vi "Configure Tester Dialog.vi"(8 "error in":errorcluster, 11 "Potting Procedure In":refnum<class "Potting Procedure.lvclass">) -> (0 "error out":errorcluster, 2 "Canceled":bool, 3 "Potting Procedure Out":refnum<class "Potting Procedure.lvclass">)   [LabVIEW 2011]
uses:
  UI typedefs/Chuck Control.ctl
  UI typedefs/Chuck Slot Control.ctl
  Procedure Classes/Potting Procedure/Potting Procedure.lvclass
  Shared Components/WorkTable Class/WorkTable Class.lvclass
  Procedure Classes/Potting Procedure/Type Definitions/Configure Tester.ctl
panel:
  in  "Module Chuck 5":T1
  in  "Module Chuck 4":T1
  in  "Module Chuck 3":T1
  in  "Module Chuck 2":T1
  in  "Module Chuck 1":T1
  in  "OK Button":bool
  in  "Cancel Button":bool
  # "Click inside the boxes to indicate whether\na slot is populated.\n\nFor each populated chuck enter the serial\nnumber in the provided text field."
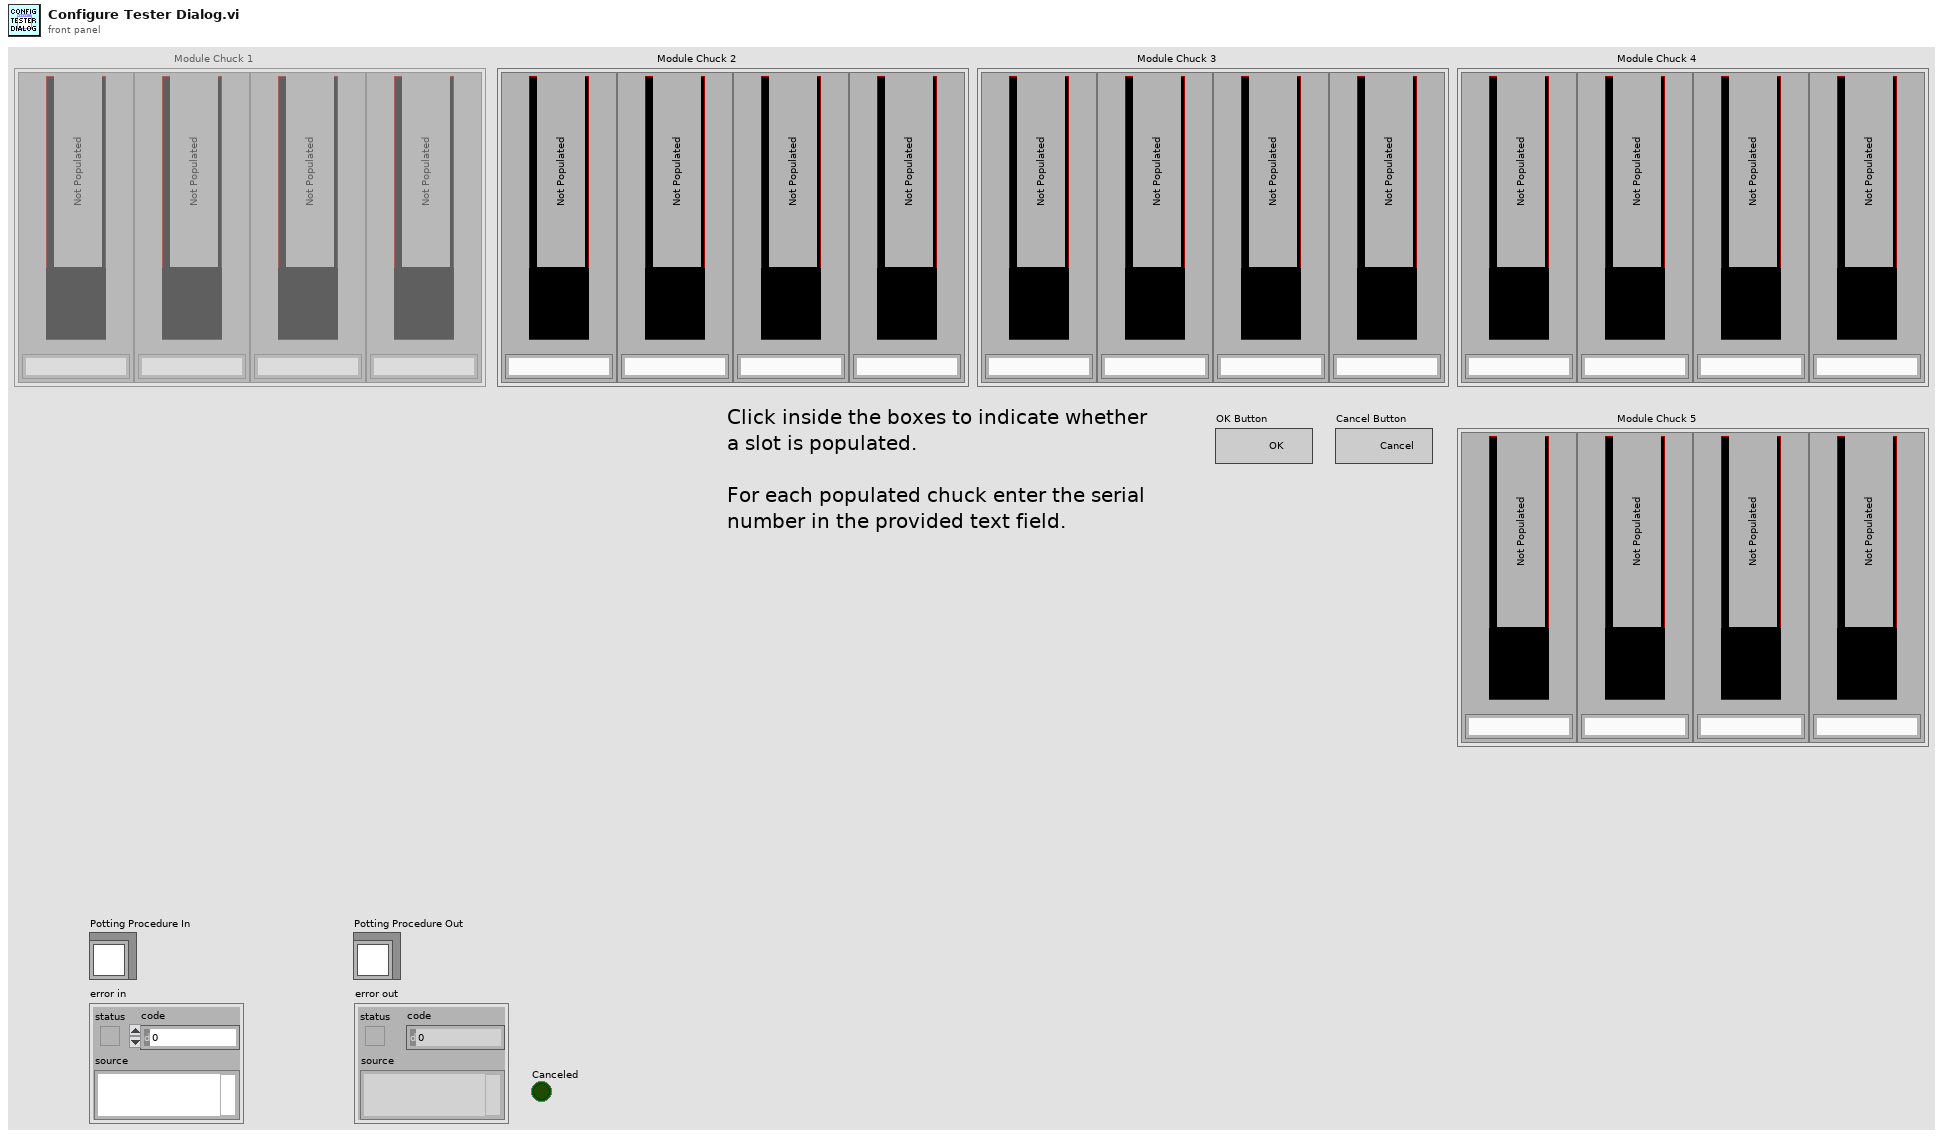
[diagram p1: front panel]
types:
  T1 = typedef "Chuck Control.ctl" = cluster{"Slot 1":T2, "Slot 2":T2, "Slot 3":T2, "Slot 4":T2}
  T2 = typedef "Chuck Slot Control.ctl" = cluster{"Slot Populated":bool, "S/N":string}
  T3 = enum8{"Enabled", "Disabled", "Disabled and Grayed Out"}
  T4 = enum16{"Empty", "Unglued", "Stamped", "PartOnTop", "Weighted", "Unpotted", "Potted"}
  T5 = typedef "Worktable_Module Slot.ctl" = cluster{"Slot State":enum16{"Empty", "Unglued", "Stamped", "PartOnTop", "Weighted", "Unpotted", "Potted"}, "BBM Type":enum16{"None", "BBM", "GlassSlide"}, "HDI Type":enum16{"None", "HDI", "Polyimide"}, "Vacuum Channel":u8, "Location/Orientation BBM":T6, "Location/Orientation HDI":T6, "S/N":string}
  T6 = typedef "Position_Orientation.ctl" = cluster{"Center":refnum<class "Vec3d Class.lvclass">, "Orientation":refnum<class "Orient3d Class.lvclass">}
  T7 = typedef "Configure Tester.ctl" = cluster{"Has Been Run?":bool}
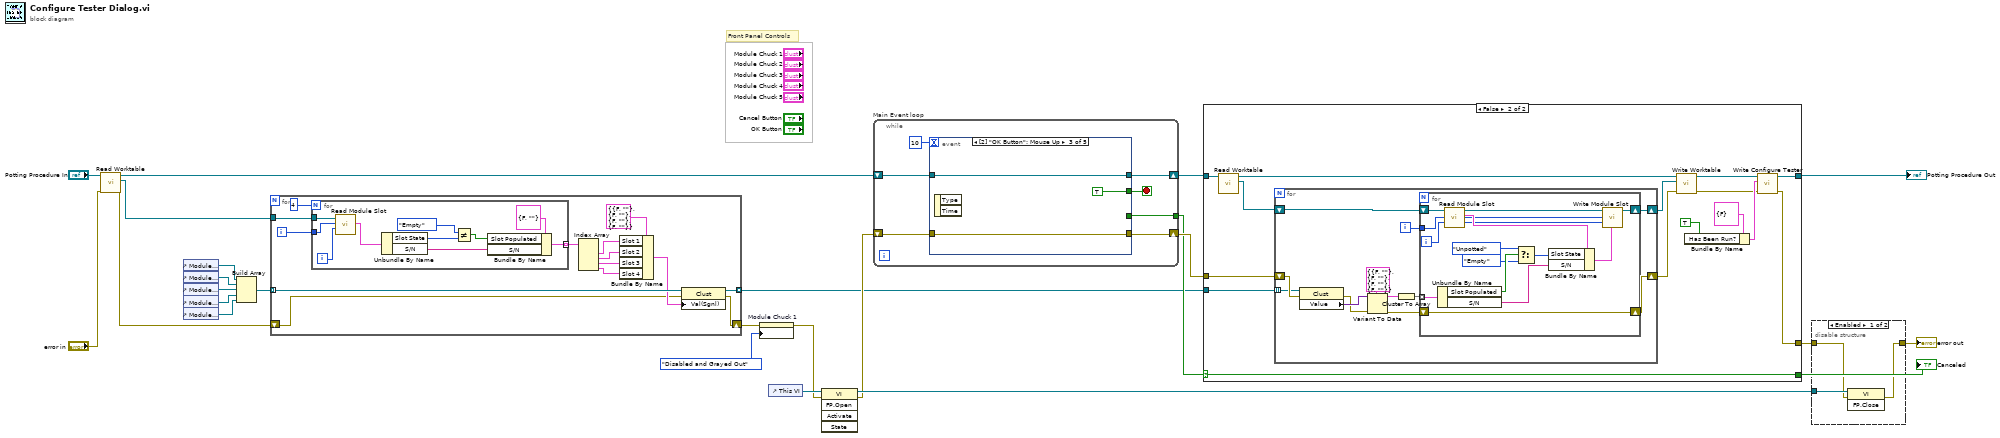
[diagram p0: block diagram]
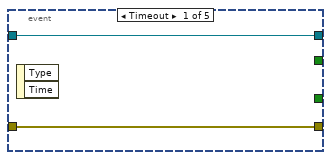
[diagram p4: hidden frame]
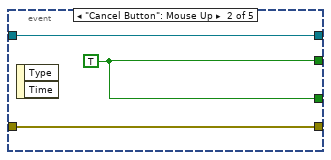
[diagram p5: hidden frame]
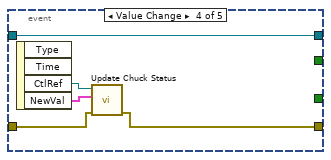
[diagram p6: hidden frame]
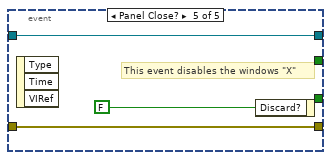
[diagram p7: hidden frame]
diagram:
  # "Front Panel Controls"
  n1 = call-dynamic "Read Worktable.vi"("error in"="error in", "Potting Procedure in"="Potting Procedure In") -> ("error out"=w4:errorcluster, "WorkTable out"=w5:refnum<class "WorkTable Class.lvclass">, "Potting Procedure out"=w17:refnum<class "Potting Procedure.lvclass">)  [unwired: 7 in]
  n2 = control-ref of="Module Chuck 1"() -> (w10:refnum<vi>)
  n3 = control-ref of="Module Chuck 2"() -> (w9:refnum<vi>)
  n4 = control-ref of="Module Chuck 3"() -> (w8:refnum<vi>)
  n5 = control-ref of="Module Chuck 4"() -> (w7:refnum<vi>)
  n6 = control-ref of="Module Chuck 5"() -> (w6:refnum<vi>)
  n7 = Build Array(w10, w9, w8, w7, w6) -> (w2:refnum<vi>[])
  n8 = for {
    tunnel: w2 -> [w32] mode=indexing
    shift-right: [w30] -> w3
    shift-left: w4 -> [w29]
    tunnel: w5 -> [w27]
    tunnel: [w28] -> w1 mode=indexing
    i -> [w26]
    n9 = for {
      N: 4 -> [_]
      tunnel: [w46] -> w37 mode=indexing
      tunnel: w27 -> [w43]
      tunnel: w26 -> [w41]
      i -> [w42]
      n10 = call-dynamic "Read Module Slot.vi"("slot"=w42, "chuck"=w41, "WorkTable in"=w43) -> ("Module Slot"=w40:T5)  [unwired: 6 in, 2 out]
      n11 = Unbundle By Name(w40) -> ("Slot State"=w45:T4, "S/N"=w44:string)
      n12 = Not Equal?(x=T4."Empty" ("BBM Slot State"), y=w45) -> (x != y?=w47:bool)
      n13 = Bundle By Name(cluster=T2 {"Slot Populated"=FALSE, "S/N"=""} ("Slot 1"), "Slot Populated"=w47, "S/N"=w44) -> (w46:T2)
    }
    n14 = Index Array(array=w37) -> (element #1=w36:T2, element #2=w35:T2, element #3=w34:T2, element #4=w33:T2)  [unwired: 4 in]
    n15 = Bundle By Name(cluster=T1 {"Slot 1"={"Slot Populated"=FALSE, "S/N"=""}, "Slot 2"={"Slot Populated"=FALSE, "S/N"=""}, "Slot 3"={"Slot Populated"=FALSE, "S/N"=""}, "Slot 4"={"Slot Populated"=FALSE, "S/N"=""}} ("BBM Chuck 1"), "Slot 1"=w36, "Slot 2"=w35, "Slot 3"=w34, "Slot 4"=w33) -> (w31:T1)
    n16 = property class="Clust"(reference=w32, error in=w29, "Val(Sgnl)"=w31) -> (reference out=w28:refnum<vi>, error out=w30:errorcluster)
  }
  n17 = property on="Module Chuck 1" class="Clust"(error in=w3, "DisabledEnum"=T3."Disabled and Grayed Out" ("Disabled")) -> (error out=w12:errorcluster)  [unwired: 1 in, 1 out]
  n18 = control-ref of="This VI"() -> (w25:refnum<vi>)
  n19 = invoke class="VI" method="FP.Open"(reference=w25, error in=w12) -> (reference out=w24:refnum<vi>, error out=w22:errorcluster)  [unwired: 3 in, 3 out]
  n20 = while "Main Event loop" {
    tunnel: [w52] -> w14
    shift-right: [w50] -> w20
    shift-left: w17 -> [w51]
    shift-right: [w54] -> w16
    shift-left: w22 -> [w53]
    stop <- w55 stop-if-true
    n21 = event shown="[2] \"OK Button\": Mouse Up" {
      selector: _ -> [_ _ _ _ _]
      dyn-events: _ -> [_ _ _ _ _]
      timeout: 10 -> [_ _ _ _ _]
      tunnel: [_ w60 TRUE _ _] -> w55
      tunnel: [w58 w61 w64 w65 w71] -> w54
      tunnel: w53 -> [w58 w61 w64 w68 w71]
      tunnel: [_ w60 _ _ _] -> w52
      tunnel: w51 -> [w57 w59 w62 w66 w70]
      tunnel: [w57 w59 w62 w66 w70] -> w50
      event Timeout {
        n22 = event-data() -> ()  [unwired: 1 in, 2 out]
      }
      event "Cancel Button": Mouse Up {
        w60 = TRUE
        n23 = event-data() -> ()  [unwired: 1 in, 2 out]
      }
      event "OK Button": Mouse Up {
        n24 = event-data() -> ()  [unwired: 1 in, 2 out]
      }
      event Value Change {
        n25 = event-data() -> ("CtlRef"=w69:refnum<vi>, "NewVal"=w67:T1)  [unwired: 1 in, 2 out]
        n26 = call "Update Chuck Status.vi"("error in"=w68, "Chuck Value"=w67, "Chuck Reference In"=w69) -> ("error out"=w65:errorcluster)  [unwired: 8 in]
      }
      event Panel Close? {
        # "This event disables the windows \"X\""
        n27 = event-data() -> ()  [unwired: 1 in, 3 out]
        n28 = event-data("Discard?"=FALSE) -> ()  [unwired: 1 in, 1 out]
      }
    }
  }
  n29 = case shown="False" w14 {
    selector: w14 -> [w73 w85]
    tunnel: w20 -> [w75 w84]
    tunnel: [w75 w90] -> w19
    tunnel: w16 -> [w74 w77]
    tunnel: [w74 w87] -> w15
    tunnel: [w73 w85] -> w11
    tunnel: w1 -> [_ w76]
    frame True {
    }
    frame False {
      n30 = call-dynamic "Read Worktable.vi"("Potting Procedure in"=w84) -> ("WorkTable out"=w83:refnum<class "WorkTable Class.lvclass">, "Potting Procedure out"=w82:refnum<class "Potting Procedure.lvclass">)  [unwired: 8 in, 1 out]
      n31 = for {
        shift-right: [w97] -> w78
        shift-left: w83 -> [w99]
        shift-right: [w95] -> w79
        shift-left: w77 -> [w94]
        tunnel: w76 -> [w91] mode=indexing
        i -> [w98]
        n32 = property class="Clust"(reference=w91, error in=w94) -> (error out=w92:errorcluster, "Value"=w93:variant)  [unwired: 1 out]
        n33 = Variant To Data(error in=w92, type=T1 {"Slot 1"={"Slot Populated"=FALSE, "S/N"=""}, "Slot 2"={"Slot Populated"=FALSE, "S/N"=""}, "Slot 3"={"Slot Populated"=FALSE, "S/N"=""}, "Slot 4"={"Slot Populated"=FALSE, "S/N"=""}} ("BBM Chuck 1"), Variant=w93) -> (data=w101:T1, error out=w96:errorcluster)
        n34 = Cluster To Array(cluster=w101) -> (array=w100:T2[])
        n35 = for {
          tunnel: w100 -> [w116] mode=indexing
          tunnel: w98 -> [w108]
          shift-right: [w106] -> w97
          shift-left: w99 -> [w104]
          shift-right: [w105] -> w95
          shift-left: w96 -> [w105]
          i -> [w109]
          n36 = Unbundle By Name(w116) -> ("Slot Populated"=w114:bool, "S/N"=w115:string)
          n37 = call-dynamic "Read Module Slot.vi"("slot"=w109, "chuck"=w108, "WorkTable in"=w104) -> ("Module Slot"=w110:T5, "WorkTable out"=w103:refnum<class "WorkTable Class.lvclass">)  [unwired: 6 in, 1 out]
          n38 = Select(t=T4."Unpotted" ("BBM Slot State"), s=w114, f=T4."Empty" ("BBM Slot State")) -> (s? t:f=w111:T4)
          n39 = Bundle By Name(cluster=w110, "Slot State"=w111, "S/N"=w115) -> (w107:T5)
          n40 = call-dynamic "Write Module Slot.vi"("Module Slot"=w107, "slot"=w109, "chuck"=w108, "WorkTable in"=w103) -> ("WorkTable out"=w106:refnum<class "WorkTable Class.lvclass">)  [unwired: 6 in, 1 out]
        }
      }
      n41 = call-dynamic "Write Worktable.vi"("error in"=w79, "WorkTable in"=w78, "Potting Procedure in"=w82) -> ("error out"=w80:errorcluster, "Potting Procedure out"=w81:refnum<class "Potting Procedure.lvclass">)  [unwired: 7 in]
      n42 = Bundle By Name(cluster=T7 {"Has Been Run?"=FALSE} ("Configure Tester"), "Has Been Run?"=TRUE) -> (w88:T7)
      n43 = call-dynamic "Write Configure Tester.vi"("error in (no error)"=w80, "Configure Tester"=w88, "Potting Procedure in"=w81) -> ("error out"=w87:errorcluster, "Potting Procedure out"=w90:refnum<class "Potting Procedure.lvclass">)  [unwired: 7 in]
    }
  }
  "Canceled" <- w11
  "Potting Procedure Out" <- w19
  n44 = disable-structure shown="Enabled" {
    disable-tunnel: w24 -> [w119 _]
    disable-tunnel: [w118 w120] -> w23
    disable-tunnel: w15 -> [w117 w120]
    frame Enabled {
      n45 = invoke class="VI" method="FP.Close"(reference=w119, error in=w117) -> (error out=w118:errorcluster)  [unwired: 1 in, 2 out]
    }
    frame Disabled {
    }
  }
  "error out" <- w23
